vi "メイン.vi"() -> (2 "測定周期/ms":dbl, 3 "値転記用配列":T2[](array[typedef]))   [LabVIEW 2021] (continued)
                          # "csv作成の為表へクラスタ(実測値)書き込み"
                          # "⑤"
                          # "③"
                          # "④"
                          n2701 = local read "メインON/OFF_\n設定 10"() -> (w4992:T1)
                          n2702 = Unbundle By Name(w4992) -> ("使用ON/OFF"=w4988:bool)
                          n2703 = control-ref of="前回値転記用配列"() -> (w4986:refnum<vi>)
                          n2704 = local read "メイン設定_設定 10"() -> (w4993:T2)
                          n2705 = call "メイン_測定値配列_CSV転記サブ.vi"("メイン設定_設定入力"=w4993, "ループ反復数値入力"=w4990, "実測設定項目"=w4991, "使用ON/OFF"=w4988, "前回値転記用配列"=w4986) -> ("ループ反復数値出力"=w4989:i32, "メイン設定_設定出力"=w4987:T2)  [unwired: 5 in]
                          n2706 = local write "メイン設定_設定 10"(w4987) -> ()
                          n2707 = Add(x=11, y=w4989) -> (x+y=w4982:i32)
                          n2708 = Add(x=w4989, y=12) -> (x+y=w4980:i32)
                          n2709 = local read "csv作成表"() -> (w4976:string[][])
                          n2710 = Unbundle By Name(w4987) -> ("実測値(MAX)"=w4983:string, "実測値(MIN)"=w4984:string)
                          n2711 = Replace Array Subset(array=w4976, new element #1=w4983, index (row) #1=w4981, index (col) #1=w4982, new element #2=w4984, index (row) #2=w4981, index (col) #2=w4980) -> (w4978:string[][])
                          n2712 = Select(t=w4978, s=w4988, f=w4976) -> (s? t:f=w4979:string[][])
                          n2713 = local write "csv作成表"(w4979) -> ()
                        }
                        frame 10 {
                          w4999 = 2
                          # "B"
                          # "A"
                          # "csv作成の為表へクラスタ(実測値)書き込み"
                          # "⑤"
                          # "③"
                          # "④"
                          n2714 = local read "メインON/OFF_\n設定 11"() -> (w5010:T1)
                          n2715 = Unbundle By Name(w5010) -> ("使用ON/OFF"=w5006:bool)
                          n2716 = control-ref of="前回値転記用配列"() -> (w5004:refnum<vi>)
                          n2717 = local read "メイン設定_設定 11"() -> (w5011:T2)
                          n2718 = call "メイン_測定値配列_CSV転記サブ.vi"("メイン設定_設定入力"=w5011, "ループ反復数値入力"=w5008, "実測設定項目"=w5009, "使用ON/OFF"=w5006, "前回値転記用配列"=w5004) -> ("ループ反復数値出力"=w5007:i32, "メイン設定_設定出力"=w5005:T2)  [unwired: 5 in]
                          n2719 = local write "メイン設定_設定 11"(w5005) -> ()
                          n2720 = Add(x=12, y=w5007) -> (x+y=w5000:i32)
                          n2721 = Add(x=w5007, y=13) -> (x+y=w4998:i32)
                          n2722 = local read "csv作成表"() -> (w4994:string[][])
                          n2723 = Unbundle By Name(w5005) -> ("実測値(MAX)"=w5001:string, "実測値(MIN)"=w5002:string)
                          n2724 = Replace Array Subset(array=w4994, new element #1=w5001, index (row) #1=w4999, index (col) #1=w5000, new element #2=w5002, index (row) #2=w4999, index (col) #2=w4998) -> (w4996:string[][])
                          n2725 = Select(t=w4996, s=w5006, f=w4994) -> (s? t:f=w4997:string[][])
                          n2726 = local write "csv作成表"(w4997) -> ()
                        }
                        frame 11 {
                          w5017 = 2
                          # "B"
                          # "A"
                          # "csv作成の為表へクラスタ(実測値)書き込み"
                          # "⑤"
                          # "③"
                          # "④"
                          n2727 = local read "メインON/OFF_\n設定 12"() -> (w5028:T1)
                          n2728 = Unbundle By Name(w5028) -> ("使用ON/OFF"=w5024:bool)
                          n2729 = control-ref of="前回値転記用配列"() -> (w5022:refnum<vi>)
                          n2730 = local read "メイン設定_設定 12"() -> (w5029:T2)
                          n2731 = call "メイン_測定値配列_CSV転記サブ.vi"("メイン設定_設定入力"=w5029, "ループ反復数値入力"=w5026, "実測設定項目"=w5027, "使用ON/OFF"=w5024, "前回値転記用配列"=w5022) -> ("ループ反復数値出力"=w5025:i32, "メイン設定_設定出力"=w5023:T2)  [unwired: 5 in]
                          n2732 = local write "メイン設定_設定 12"(w5023) -> ()
                          n2733 = Add(x=13, y=w5025) -> (x+y=w5018:i32)
                          n2734 = Add(x=w5025, y=14) -> (x+y=w5016:i32)
                          n2735 = local read "csv作成表"() -> (w5012:string[][])
                          n2736 = Unbundle By Name(w5023) -> ("実測値(MAX)"=w5019:string, "実測値(MIN)"=w5020:string)
                          n2737 = Replace Array Subset(array=w5012, new element #1=w5019, index (row) #1=w5017, index (col) #1=w5018, new element #2=w5020, index (row) #2=w5017, index (col) #2=w5016) -> (w5014:string[][])
                          n2738 = Select(t=w5014, s=w5024, f=w5012) -> (s? t:f=w5015:string[][])
                          n2739 = local write "csv作成表"(w5015) -> ()
                        }
                      }
                    }
                  }
                }
                n2740 = local write "値転記用配列"(w4786) -> ()
                n2741 = flat-sequence {
                  tunnel: [w4801] -> w4787
                  tunnel: w4786 -> [w4801]
                  frame #0 {
                    w4796 = T9 {"Horizontal"=-51, "Vertical"=360} ("座標 5")
                    n2742 = control-ref of="このVI"() -> (w4797:refnum<vi>)
                    n2743 = property on="ペーン 2" class="Pane"("Origin"=w4796) -> ()  [unwired: 2 in, 2 out]
                    n2744 = property on="ペーン 2" class="Pane"("Origin"=w4796) -> ()  [unwired: 2 in, 2 out]
                    n2745 = control-ref of="このVI"() -> (w4799:refnum<vi>)
                    n2746 = Unbundle(w4796) -> ("Vertical"=w4798:i16)  [unwired: 1 out]
                    n2747 = Unbundle(w4796) -> ("Vertical"=w4800:i16)  [unwired: 1 out]
                    n2748 = call "メイン_装飾移動サブ.vi"("Y軸座標入力"=w4798, "VI入力"=w4797) -> ()  [unwired: 10 in]
                    n2749 = call "メイン_装飾枠移動サブ.vi"("Y軸座標入力"=w4800, "VI入力"=w4799) -> ()  [unwired: 10 in]
                  }
                }
              }
              frame #1 {
                w5031 = T8."Enabled" ("無効")
                # "⑪ボタンの無効解除"
                n2750 = for {
                  N: 12 -> [_]
                  tunnel: w5031 -> [w5034]
                  i -> [w5035]
                  n2751 = case shown="11" w5035 {
                    tunnel: w5034 -> [w5036 w5037 w5038 w5039 w5040 w5041 w5042 w5043 w5044 w5045 w5046 w5047]
                    frame 0, Default {
                      n2752 = property on="メイン測定ボタン_単発 1" class="Bool (指定)"("DisabledEnum"=w5036) -> ()  [unwired: 2 in, 2 out]
                      n2753 = property on="メイン測定ボタン_連続 1" class="Bool (指定)"("DisabledEnum"=w5036) -> ()  [unwired: 2 in, 2 out]
                    }
                    frame 1 {
                      n2754 = property on="メイン測定ボタン_単発 2" class="Bool (指定)"("DisabledEnum"=w5037) -> ()  [unwired: 2 in, 2 out]
                      n2755 = property on="メイン測定ボタン_連続 2" class="Bool (指定)"("DisabledEnum"=w5037) -> ()  [unwired: 2 in, 2 out]
                    }
                    frame 2 {
                      n2756 = property on="メイン測定ボタン_単発 3" class="Bool (指定)"("DisabledEnum"=w5038) -> ()  [unwired: 2 in, 2 out]
                      n2757 = property on="メイン測定ボタン_連続 3" class="Bool (指定)"("DisabledEnum"=w5038) -> ()  [unwired: 2 in, 2 out]
                    }
                    frame 3 {
                      n2758 = property on="メイン測定ボタン_単発 4" class="Bool (指定)"("DisabledEnum"=w5039) -> ()  [unwired: 2 in, 2 out]
                      n2759 = property on="メイン測定ボタン_連続 4" class="Bool (指定)"("DisabledEnum"=w5039) -> ()  [unwired: 2 in, 2 out]
                    }
                    frame 4 {
                      n2760 = property on="メイン測定ボタン_単発 5" class="Bool (指定)"("DisabledEnum"=w5040) -> ()  [unwired: 2 in, 2 out]
                      n2761 = property on="メイン測定ボタン_連続 5" class="Bool (指定)"("DisabledEnum"=w5040) -> ()  [unwired: 2 in, 2 out]
                    }
                    frame 5 {
                      n2762 = property on="メイン測定ボタン_連続 6" class="Bool (指定)"("DisabledEnum"=w5041) -> ()  [unwired: 2 in, 2 out]
                      n2763 = property on="メイン測定ボタン_単発 6" class="Bool (指定)"("DisabledEnum"=w5041) -> ()  [unwired: 2 in, 2 out]
                    }
                    frame 6 {
                      n2764 = property on="メイン測定ボタン_連続 7" class="Bool (指定)"("DisabledEnum"=w5042) -> ()  [unwired: 2 in, 2 out]
                      n2765 = property on="メイン測定ボタン_単発 7" class="Bool (指定)"("DisabledEnum"=w5042) -> ()  [unwired: 2 in, 2 out]
                    }
                    frame 7 {
                      n2766 = property on="メイン測定ボタン_単発 8" class="Bool (指定)"("DisabledEnum"=w5043) -> ()  [unwired: 2 in, 2 out]
                      n2767 = property on="メイン測定ボタン_連続 8" class="Bool (指定)"("DisabledEnum"=w5043) -> ()  [unwired: 2 in, 2 out]
                    }
                    frame 8 {
                      n2768 = property on="メイン測定ボタン_単発 9" class="Bool (指定)"("DisabledEnum"=w5044) -> ()  [unwired: 2 in, 2 out]
                      n2769 = property on="メイン測定ボタン_連続 9" class="Bool (指定)"("DisabledEnum"=w5044) -> ()  [unwired: 2 in, 2 out]
                    }
                    frame 9 {
                      n2770 = property on="メイン測定ボタン_単発 10" class="Bool (指定)"("DisabledEnum"=w5045) -> ()  [unwired: 2 in, 2 out]
                      n2771 = property on="メイン測定ボタン_連続 10" class="Bool (指定)"("DisabledEnum"=w5045) -> ()  [unwired: 2 in, 2 out]
                    }
                    frame 10 {
                      n2772 = property on="メイン測定ボタン_単発 11" class="Bool (指定)"("DisabledEnum"=w5046) -> ()  [unwired: 2 in, 2 out]
                      n2773 = property on="メイン測定ボタン_連続 11" class="Bool (指定)"("DisabledEnum"=w5046) -> ()  [unwired: 2 in, 2 out]
                    }
                    frame 11 {
                      n2774 = property on="メイン測定ボタン_連続 12" class="Bool (指定)"("DisabledEnum"=w5047) -> ()  [unwired: 2 in, 2 out]
                      n2775 = property on="メイン測定ボタン_単発 12" class="Bool (指定)"("DisabledEnum"=w5047) -> ()  [unwired: 2 in, 2 out]
                    }
                  }
                }
                n2776 = local write "測定新値\nリセット用 6"(TRUE) -> ()
                n2777 = property on="TOPページへ" class="Bool"("DisabledEnum"=w5031) -> ()  [unwired: 2 in, 2 out]
                n2778 = property on="保存して終了" class="Bool"("DisabledEnum"=w5031) -> ()  [unwired: 2 in, 2 out]
                n2779 = property on="保存せずに" class="Bool"("DisabledEnum"=w5031) -> ()  [unwired: 2 in, 2 out]
              }
            }
          }
          frame True {
          }
        }
      }
      frame "測定7" {
        # "⑦"
        # "項目別のボタンで測定を行う為、項目分必要"
        n2780 = local read "測定旧値 7"() -> (w5051:bool)
        n2781 = case shown="FALSE" w5051 {
          tunnel: w5049 -> [w5054 w5317]
          tunnel: [w5053 w5317] -> w5050
          frame False {
            n2782 = flat-sequence {
              tunnel: w5054 -> [w5064]
              tunnel: [w5056] -> w5052
              tunnel: [w5302] -> w5053
              tunnel: w5052 -> [w5302]
              frame #0 {
                # "※複製コピー時変更する項目\n①②\nローカル変数\n\n入れ子のケースストラクチャ\"2\"を複製\n\n0～数だけ変更する\n③④⑤\nローカル変数\n\n※AB\n行番号の変更をする必要がある\n\n--------------------------------\nこの後イベントストラクチャ複製する\n--------------------------------\nイベントストラクチャ複製後\n\n⑦⑧\nローカル変数\n⑨\n装飾体の位置設定\n-51は固定\n前ケースの数値+72\n⑩\n測定新値リセット用\nのボタンが複製されているので、\nフロントパネルを整理する\n⑪\nプロパティノード\nボタンの無効解除クリア以外全てのボタン対象"
                # "実測完了の簡易疑似コード\n\n1)測定モードが単発・連続、多点かで転記する配列を変える\n2)値転記用配列へ転記\n\nここからゲージ分を繰り返す必要がある\n\n3)配列0を取り出す\n4)配列0のポートNoを取り出す\n5)メイン測定_設定配列(測定1の対象配列)のポートNoと比較\n6)同じだったら処理をする。違ったら何もしない\n7)同じだったら配列0のメインON/OFF_設定1の使用ON/OFFがTrueかFalseか\nFlaseだったら前回値転記用配列から前回の値をメイン設定_設定へ転記\nTrueだったらメイン設定_設定の測定モードから\n0単発、1連続、3多点\nの処理を行う\n8)測定値をメイン設定_設定へ転記したら、前回転記用配列へ転記する"
                # "⑨"
                # "⑧"
                # "②"
                # "グループNO(表示上はポートNo)が同じだったら値を転記する\n\n測定した配列のグループNOと値転記用配列の他の指標グループNOを比較する\n＝だったら、対象の配列のON/OFFボタンがTrueか確認し、\nTrueだったら、測定モードによって、値かMAX、MINの数値を転記する\n\nグループNOが同じでなければ、転記しない(何もしない)"
                # "まず値転記用配列に測定の値を転記"
                # "実測定画面vi動作"
                n2783 = local read "メイン設定_設定 7"() -> (w5059:T2)
                n2784 = local read "測定新値 7"() -> (→"測定新値\nリセット用 7":bool)
                n2785 = local read "測定周期/ms"() -> (w5057:dbl)
                n2786 = Unbundle By Name(w5059) -> ("測定モード"=w5060:u16)
                n2787 = call "実測定画面.vi"("実測設定項目配列_\nメインからの転記"=w5064, "測定周期/ms_制御器"=w5057) -> ("実測設定項目配列_\nゲージIOへ転記用"=w5062:T2[], "実測設定項目配列_\n多点測定メイン転記用"=w5061:T2[])  [unwired: 11 in, 1 out]
                n2788 = case shown="1" w5060 {
                  tunnel: w5062 -> [w5071 w5072 _]
                  tunnel: [w5071 w5072 w5073] -> w5055
                  tunnel: w5061 -> [_ _ w5073]
                  frame 0, Default {
                  }
                  frame 1 {
                  }
                  frame 2 {
                  }
                }
                n2789 = for {
                  N: 32 -> [_]
                  tunnel: w5055 -> [w5080]
                  i -> [w5075]
                  # "①"
                  # "※複製コピーはこのケースで行う"
                  # "32回分"
                  # "比較する固定GNO"
                  n2790 = local read "メイン設定_設定 7"() -> (w5074:T2)
                  n2791 = Index Array(array=w5080, index=w5075) -> (element=w5079:T2)
                  n2792 = Unbundle By Name(w5074) -> ("ポートNo."=w5078:dbl)
                  n2793 = Unbundle By Name(w5079) -> ("ポートNo."=w5077:dbl)
                  n2794 = Equal?(x=w5078, y=w5077) -> (x = y?=w5076:bool)
                  n2795 = case shown="TRUE" w5076 {
                    tunnel: w5079 -> [_ w5082]
                    tunnel: w5075 -> [_ w5081]
                    frame False {
                    }
                    frame True {
                      n2796 = case shown="0, デフォルト" w5081 {
                        tunnel: w5082 -> [w5098 w5116 w5134 w5152 w5170 w5188 w5206 w5224 w5242 w5260 w5278 w5296]
                        tunnel: w5081 -> [w5097 w5115 w5133 w5151 w5169 w5187 w5205 w5223 w5241 w5259 w5277 w5295]
                        frame 0, Default {
                          w5088 = 2
                          # "B"
                          # "A"
                          # "csv作成の為表へクラスタ(実測値)書き込み"
                          # "⑤"
                          # "③"
                          # "④"
                          n2797 = local read "メインON/OFF_\n設定 1"() -> (w5099:T1)
                          n2798 = Unbundle By Name(w5099) -> ("使用ON/OFF"=w5095:bool)
                          n2799 = control-ref of="前回値転記用配列"() -> (w5093:refnum<vi>)
                          n2800 = local read "メイン設定_設定 1"() -> (w5100:T2)
                          n2801 = call "メイン_測定値配列_CSV転記サブ.vi"("メイン設定_設定入力"=w5100, "ループ反復数値入力"=w5097, "実測設定項目"=w5098, "使用ON/OFF"=w5095, "前回値転記用配列"=w5093) -> ("ループ反復数値出力"=w5096:i32, "メイン設定_設定出力"=w5094:T2)  [unwired: 5 in]
                          n2802 = local write "メイン設定_設定 1"(w5094) -> ()
                          n2803 = Add(x=2, y=w5096) -> (x+y=w5089:i32)
                          n2804 = Add(x=w5096, y=3) -> (x+y=w5087:i32)
                          n2805 = local read "csv作成表"() -> (w5083:string[][])
                          n2806 = Unbundle By Name(w5094) -> ("実測値(MAX)"=w5090:string, "実測値(MIN)"=w5091:string)
                          n2807 = Replace Array Subset(array=w5083, new element #1=w5090, index (row) #1=w5088, index (col) #1=w5089, new element #2=w5091, index (row) #2=w5088, index (col) #2=w5087) -> (w5085:string[][])
                          n2808 = Select(t=w5085, s=w5095, f=w5083) -> (s? t:f=w5086:string[][])
                          n2809 = local write "csv作成表"(w5086) -> ()
                        }
                        frame 1 {
                          w5106 = 2
                          # "B"
                          # "A"
                          # "csv作成の為表へクラスタ(実測値)書き込み"
                          # "⑤"
                          # "③"
                          # "④"
                          n2810 = local read "メインON/OFF_\n設定 2"() -> (w5117:T1)
                          n2811 = Unbundle By Name(w5117) -> ("使用ON/OFF"=w5113:bool)
                          n2812 = control-ref of="前回値転記用配列"() -> (w5111:refnum<vi>)
                          n2813 = local read "メイン設定_設定 2"() -> (w5118:T2)
                          n2814 = call "メイン_測定値配列_CSV転記サブ.vi"("メイン設定_設定入力"=w5118, "ループ反復数値入力"=w5115, "実測設定項目"=w5116, "使用ON/OFF"=w5113, "前回値転記用配列"=w5111) -> ("ループ反復数値出力"=w5114:i32, "メイン設定_設定出力"=w5112:T2)  [unwired: 5 in]
                          n2815 = local write "メイン設定_設定 2"(w5112) -> ()
                          n2816 = Add(x=3, y=w5114) -> (x+y=w5107:i32)
                          n2817 = Add(x=w5114, y=4) -> (x+y=w5105:i32)
                          n2818 = local read "csv作成表"() -> (w5101:string[][])
                          n2819 = Unbundle By Name(w5112) -> ("実測値(MAX)"=w5108:string, "実測値(MIN)"=w5109:string)
                          n2820 = Replace Array Subset(array=w5101, new element #1=w5108, index (row) #1=w5106, index (col) #1=w5107, new element #2=w5109, index (row) #2=w5106, index (col) #2=w5105) -> (w5103:string[][])
                          n2821 = Select(t=w5103, s=w5113, f=w5101) -> (s? t:f=w5104:string[][])
                          n2822 = local write "csv作成表"(w5104) -> ()
                        }
                        frame 2 {
                          w5124 = 2
                          # "B"
                          # "A"
                          # "csv作成の為表へクラスタ(実測値)書き込み"
                          # "⑤"
                          # "③"
                          # "④"
                          n2823 = local read "メインON/OFF_\n設定 3"() -> (w5135:T1)
                          n2824 = Unbundle By Name(w5135) -> ("使用ON/OFF"=w5131:bool)
                          n2825 = control-ref of="前回値転記用配列"() -> (w5129:refnum<vi>)
                          n2826 = local read "メイン設定_設定 3"() -> (w5136:T2)
                          n2827 = call "メイン_測定値配列_CSV転記サブ.vi"("メイン設定_設定入力"=w5136, "ループ反復数値入力"=w5133, "実測設定項目"=w5134, "使用ON/OFF"=w5131, "前回値転記用配列"=w5129) -> ("ループ反復数値出力"=w5132:i32, "メイン設定_設定出力"=w5130:T2)  [unwired: 5 in]
                          n2828 = local write "メイン設定_設定 3"(w5130) -> ()
                          n2829 = Add(x=4, y=w5132) -> (x+y=w5125:i32)
                          n2830 = Add(x=w5132, y=5) -> (x+y=w5123:i32)
                          n2831 = local read "csv作成表"() -> (w5119:string[][])
                          n2832 = Unbundle By Name(w5130) -> ("実測値(MAX)"=w5126:string, "実測値(MIN)"=w5127:string)
                          n2833 = Replace Array Subset(array=w5119, new element #1=w5126, index (row) #1=w5124, index (col) #1=w5125, new element #2=w5127, index (row) #2=w5124, index (col) #2=w5123) -> (w5121:string[][])
                          n2834 = Select(t=w5121, s=w5131, f=w5119) -> (s? t:f=w5122:string[][])
                          n2835 = local write "csv作成表"(w5122) -> ()
                        }
                        frame 3 {
                          w5142 = 2
                          # "B"
                          # "A"
                          # "csv作成の為表へクラスタ(実測値)書き込み"
                          # "⑤"
                          # "③"
                          # "④"
                          n2836 = local read "メインON/OFF_\n設定 4"() -> (w5153:T1)
                          n2837 = Unbundle By Name(w5153) -> ("使用ON/OFF"=w5149:bool)
                          n2838 = control-ref of="前回値転記用配列"() -> (w5147:refnum<vi>)
                          n2839 = local read "メイン設定_設定 4"() -> (w5154:T2)
                          n2840 = call "メイン_測定値配列_CSV転記サブ.vi"("メイン設定_設定入力"=w5154, "ループ反復数値入力"=w5151, "実測設定項目"=w5152, "使用ON/OFF"=w5149, "前回値転記用配列"=w5147) -> ("ループ反復数値出力"=w5150:i32, "メイン設定_設定出力"=w5148:T2)  [unwired: 5 in]
                          n2841 = local write "メイン設定_設定 4"(w5148) -> ()
                          n2842 = Add(x=5, y=w5150) -> (x+y=w5143:i32)
                          n2843 = Add(x=w5150, y=6) -> (x+y=w5141:i32)
                          n2844 = local read "csv作成表"() -> (w5137:string[][])
                          n2845 = Unbundle By Name(w5148) -> ("実測値(MAX)"=w5144:string, "実測値(MIN)"=w5145:string)
                          n2846 = Replace Array Subset(array=w5137, new element #1=w5144, index (row) #1=w5142, index (col) #1=w5143, new element #2=w5145, index (row) #2=w5142, index (col) #2=w5141) -> (w5139:string[][])
                          n2847 = Select(t=w5139, s=w5149, f=w5137) -> (s? t:f=w5140:string[][])
                          n2848 = local write "csv作成表"(w5140) -> ()
                        }
                        frame 4 {
                          w5160 = 2
                          # "B"
                          # "A"
                          # "csv作成の為表へクラスタ(実測値)書き込み"
                          # "⑤"
                          # "③"
                          # "④"
                          n2849 = local read "メインON/OFF_\n設定 5"() -> (w5171:T1)
                          n2850 = Unbundle By Name(w5171) -> ("使用ON/OFF"=w5167:bool)
                          n2851 = control-ref of="前回値転記用配列"() -> (w5165:refnum<vi>)
                          n2852 = local read "メイン設定_設定 5"() -> (w5172:T2)
                          n2853 = call "メイン_測定値配列_CSV転記サブ.vi"("メイン設定_設定入力"=w5172, "ループ反復数値入力"=w5169, "実測設定項目"=w5170, "使用ON/OFF"=w5167, "前回値転記用配列"=w5165) -> ("ループ反復数値出力"=w5168:i32, "メイン設定_設定出力"=w5166:T2)  [unwired: 5 in]
                          n2854 = local write "メイン設定_設定 5"(w5166) -> ()
                          n2855 = Add(x=6, y=w5168) -> (x+y=w5161:i32)
                          n2856 = Add(x=w5168, y=7) -> (x+y=w5159:i32)
                          n2857 = local read "csv作成表"() -> (w5155:string[][])
                          n2858 = Unbundle By Name(w5166) -> ("実測値(MAX)"=w5162:string, "実測値(MIN)"=w5163:string)
                          n2859 = Replace Array Subset(array=w5155, new element #1=w5162, index (row) #1=w5160, index (col) #1=w5161, new element #2=w5163, index (row) #2=w5160, index (col) #2=w5159) -> (w5157:string[][])
                          n2860 = Select(t=w5157, s=w5167, f=w5155) -> (s? t:f=w5158:string[][])
                          n2861 = local write "csv作成表"(w5158) -> ()
                        }
                        frame 5 {
                          w5178 = 2
                          # "B"
                          # "A"
                          # "csv作成の為表へクラスタ(実測値)書き込み"
                          # "⑤"
                          # "③"
                          # "④"
                          n2862 = local read "メインON/OFF_\n設定 6"() -> (w5189:T1)
                          n2863 = Unbundle By Name(w5189) -> ("使用ON/OFF"=w5185:bool)
                          n2864 = control-ref of="前回値転記用配列"() -> (w5183:refnum<vi>)
                          n2865 = local read "メイン設定_設定 6"() -> (w5190:T2)
                          n2866 = call "メイン_測定値配列_CSV転記サブ.vi"("メイン設定_設定入力"=w5190, "ループ反復数値入力"=w5187, "実測設定項目"=w5188, "使用ON/OFF"=w5185, "前回値転記用配列"=w5183) -> ("ループ反復数値出力"=w5186:i32, "メイン設定_設定出力"=w5184:T2)  [unwired: 5 in]
                          n2867 = local write "メイン設定_設定 6"(w5184) -> ()
                          n2868 = Add(x=7, y=w5186) -> (x+y=w5179:i32)
                          n2869 = Add(x=w5186, y=8) -> (x+y=w5177:i32)
                          n2870 = local read "csv作成表"() -> (w5173:string[][])
                          n2871 = Unbundle By Name(w5184) -> ("実測値(MAX)"=w5180:string, "実測値(MIN)"=w5181:string)
                          n2872 = Replace Array Subset(array=w5173, new element #1=w5180, index (row) #1=w5178, index (col) #1=w5179, new element #2=w5181, index (row) #2=w5178, index (col) #2=w5177) -> (w5175:string[][])
                          n2873 = Select(t=w5175, s=w5185, f=w5173) -> (s? t:f=w5176:string[][])
                          n2874 = local write "csv作成表"(w5176) -> ()
                        }
                        frame 6 {
                          w5196 = 2
                          # "B"
                          # "A"
                          # "csv作成の為表へクラスタ(実測値)書き込み"
                          # "⑤"
                          # "③"
                          # "④"
                          n2875 = local read "メインON/OFF_\n設定 7"() -> (w5207:T1)
                          n2876 = Unbundle By Name(w5207) -> ("使用ON/OFF"=w5203:bool)
                          n2877 = control-ref of="前回値転記用配列"() -> (w5201:refnum<vi>)
                          n2878 = local read "メイン設定_設定 7"() -> (w5208:T2)
                          n2879 = call "メイン_測定値配列_CSV転記サブ.vi"("メイン設定_設定入力"=w5208, "ループ反復数値入力"=w5205, "実測設定項目"=w5206, "使用ON/OFF"=w5203, "前回値転記用配列"=w5201) -> ("ループ反復数値出力"=w5204:i32, "メイン設定_設定出力"=w5202:T2)  [unwired: 5 in]
                          n2880 = local write "メイン設定_設定 7"(w5202) -> ()
                          n2881 = Add(x=8, y=w5204) -> (x+y=w5197:i32)
                          n2882 = Add(x=w5204, y=9) -> (x+y=w5195:i32)
                          n2883 = local read "csv作成表"() -> (w5191:string[][])
                          n2884 = Unbundle By Name(w5202) -> ("実測値(MAX)"=w5198:string, "実測値(MIN)"=w5199:string)
                          n2885 = Replace Array Subset(array=w5191, new element #1=w5198, index (row) #1=w5196, index (col) #1=w5197, new element #2=w5199, index (row) #2=w5196, index (col) #2=w5195) -> (w5193:string[][])
                          n2886 = Select(t=w5193, s=w5203, f=w5191) -> (s? t:f=w5194:string[][])
                          n2887 = local write "csv作成表"(w5194) -> ()
                        }
                        frame 7 {
                          w5214 = 2
                          # "B"
                          # "A"
                          # "csv作成の為表へクラスタ(実測値)書き込み"
                          # "⑤"
                          # "③"
                          # "④"
                          n2888 = local read "メインON/OFF_\n設定 8"() -> (w5225:T1)
                          n2889 = Unbundle By Name(w5225) -> ("使用ON/OFF"=w5221:bool)
                          n2890 = control-ref of="前回値転記用配列"() -> (w5219:refnum<vi>)
                          n2891 = local read "メイン設定_設定 8"() -> (w5226:T2)
                          n2892 = call "メイン_測定値配列_CSV転記サブ.vi"("メイン設定_設定入力"=w5226, "ループ反復数値入力"=w5223, "実測設定項目"=w5224, "使用ON/OFF"=w5221, "前回値転記用配列"=w5219) -> ("ループ反復数値出力"=w5222:i32, "メイン設定_設定出力"=w5220:T2)  [unwired: 5 in]
                          n2893 = local write "メイン設定_設定 8"(w5220) -> ()
                          n2894 = Add(x=9, y=w5222) -> (x+y=w5215:i32)
                          n2895 = Add(x=w5222, y=10) -> (x+y=w5213:i32)
                          n2896 = local read "csv作成表"() -> (w5209:string[][])
                          n2897 = Unbundle By Name(w5220) -> ("実測値(MAX)"=w5216:string, "実測値(MIN)"=w5217:string)
                          n2898 = Replace Array Subset(array=w5209, new element #1=w5216, index (row) #1=w5214, index (col) #1=w5215, new element #2=w5217, index (row) #2=w5214, index (col) #2=w5213) -> (w5211:string[][])
                          n2899 = Select(t=w5211, s=w5221, f=w5209) -> (s? t:f=w5212:string[][])
                          n2900 = local write "csv作成表"(w5212) -> ()
                        }
                        frame 8 {
                          w5232 = 2
                          # "B"
                          # "A"
                          # "csv作成の為表へクラスタ(実測値)書き込み"
                          # "⑤"
                          # "③"
                          # "④"
                          n2901 = local read "メインON/OFF_\n設定 9"() -> (w5243:T1)
                          n2902 = Unbundle By Name(w5243) -> ("使用ON/OFF"=w5239:bool)
                          n2903 = control-ref of="前回値転記用配列"() -> (w5237:refnum<vi>)
                          n2904 = local read "メイン設定_設定 9"() -> (w5244:T2)
                          n2905 = call "メイン_測定値配列_CSV転記サブ.vi"("メイン設定_設定入力"=w5244, "ループ反復数値入力"=w5241, "実測設定項目"=w5242, "使用ON/OFF"=w5239, "前回値転記用配列"=w5237) -> ("ループ反復数値出力"=w5240:i32, "メイン設定_設定出力"=w5238:T2)  [unwired: 5 in]
                          n2906 = local write "メイン設定_設定 9"(w5238) -> ()
                          n2907 = Add(x=10, y=w5240) -> (x+y=w5233:i32)
                          n2908 = Add(x=w5240, y=11) -> (x+y=w5231:i32)
                          n2909 = local read "csv作成表"() -> (w5227:string[][])
                          n2910 = Unbundle By Name(w5238) -> ("実測値(MAX)"=w5234:string, "実測値(MIN)"=w5235:string)
                          n2911 = Replace Array Subset(array=w5227, new element #1=w5234, index (row) #1=w5232, index (col) #1=w5233, new element #2=w5235, index (row) #2=w5232, index (col) #2=w5231) -> (w5229:string[][])
                          n2912 = Select(t=w5229, s=w5239, f=w5227) -> (s? t:f=w5230:string[][])
                          n2913 = local write "csv作成表"(w5230) -> ()
                        }
                        frame 9 {
                          w5250 = 2
                          # "B"
                          # "A"
                          # "csv作成の為表へクラスタ(実測値)書き込み"
                          # "⑤"
                          # "③"
                          # "④"
                          n2914 = local read "メインON/OFF_\n設定 10"() -> (w5261:T1)
                          n2915 = Unbundle By Name(w5261) -> ("使用ON/OFF"=w5257:bool)
                          n2916 = control-ref of="前回値転記用配列"() -> (w5255:refnum<vi>)
                          n2917 = local read "メイン設定_設定 10"() -> (w5262:T2)
                          n2918 = call "メイン_測定値配列_CSV転記サブ.vi"("メイン設定_設定入力"=w5262, "ループ反復数値入力"=w5259, "実測設定項目"=w5260, "使用ON/OFF"=w5257, "前回値転記用配列"=w5255) -> ("ループ反復数値出力"=w5258:i32, "メイン設定_設定出力"=w5256:T2)  [unwired: 5 in]
                          n2919 = local write "メイン設定_設定 10"(w5256) -> ()
                          n2920 = Add(x=11, y=w5258) -> (x+y=w5251:i32)
                          n2921 = Add(x=w5258, y=12) -> (x+y=w5249:i32)
                          n2922 = local read "csv作成表"() -> (w5245:string[][])
                          n2923 = Unbundle By Name(w5256) -> ("実測値(MAX)"=w5252:string, "実測値(MIN)"=w5253:string)
                          n2924 = Replace Array Subset(array=w5245, new element #1=w5252, index (row) #1=w5250, index (col) #1=w5251, new element #2=w5253, index (row) #2=w5250, index (col) #2=w5249) -> (w5247:string[][])
                          n2925 = Select(t=w5247, s=w5257, f=w5245) -> (s? t:f=w5248:string[][])
                          n2926 = local write "csv作成表"(w5248) -> ()
                        }
                        frame 10 {
                          w5268 = 2
                          # "B"
                          # "A"
                          # "csv作成の為表へクラスタ(実測値)書き込み"
                          # "⑤"
                          # "③"
                          # "④"
                          n2927 = local read "メインON/OFF_\n設定 11"() -> (w5279:T1)
                          n2928 = Unbundle By Name(w5279) -> ("使用ON/OFF"=w5275:bool)
                          n2929 = control-ref of="前回値転記用配列"() -> (w5273:refnum<vi>)
                          n2930 = local read "メイン設定_設定 11"() -> (w5280:T2)
                          n2931 = call "メイン_測定値配列_CSV転記サブ.vi"("メイン設定_設定入力"=w5280, "ループ反復数値入力"=w5277, "実測設定項目"=w5278, "使用ON/OFF"=w5275, "前回値転記用配列"=w5273) -> ("ループ反復数値出力"=w5276:i32, "メイン設定_設定出力"=w5274:T2)  [unwired: 5 in]
                          n2932 = local write "メイン設定_設定 11"(w5274) -> ()
                          n2933 = Add(x=12, y=w5276) -> (x+y=w5269:i32)
                          n2934 = Add(x=w5276, y=13) -> (x+y=w5267:i32)
                          n2935 = local read "csv作成表"() -> (w5263:string[][])
                          n2936 = Unbundle By Name(w5274) -> ("実測値(MAX)"=w5270:string, "実測値(MIN)"=w5271:string)
                          n2937 = Replace Array Subset(array=w5263, new element #1=w5270, index (row) #1=w5268, index (col) #1=w5269, new element #2=w5271, index (row) #2=w5268, index (col) #2=w5267) -> (w5265:string[][])
                          n2938 = Select(t=w5265, s=w5275, f=w5263) -> (s? t:f=w5266:string[][])
                          n2939 = local write "csv作成表"(w5266) -> ()
                        }
                        frame 11 {
                          w5286 = 2
                          # "B"
                          # "A"
                          # "csv作成の為表へクラスタ(実測値)書き込み"
                          # "⑤"
                          # "③"
                          # "④"
                          n2940 = local read "メインON/OFF_\n設定 12"() -> (w5297:T1)
                          n2941 = Unbundle By Name(w5297) -> ("使用ON/OFF"=w5293:bool)
                          n2942 = control-ref of="前回値転記用配列"() -> (w5291:refnum<vi>)
                          n2943 = local read "メイン設定_設定 12"() -> (w5298:T2)
                          n2944 = call "メイン_測定値配列_CSV転記サブ.vi"("メイン設定_設定入力"=w5298, "ループ反復数値入力"=w5295, "実測設定項目"=w5296, "使用ON/OFF"=w5293, "前回値転記用配列"=w5291) -> ("ループ反復数値出力"=w5294:i32, "メイン設定_設定出力"=w5292:T2)  [unwired: 5 in]
                          n2945 = local write "メイン設定_設定 12"(w5292) -> ()
                          n2946 = Add(x=13, y=w5294) -> (x+y=w5287:i32)
                          n2947 = Add(x=w5294, y=14) -> (x+y=w5285:i32)
                          n2948 = local read "csv作成表"() -> (w5281:string[][])
                          n2949 = Unbundle By Name(w5292) -> ("実測値(MAX)"=w5288:string, "実測値(MIN)"=w5289:string)
                          n2950 = Replace Array Subset(array=w5281, new element #1=w5288, index (row) #1=w5286, index (col) #1=w5287, new element #2=w5289, index (row) #2=w5286, index (col) #2=w5285) -> (w5283:string[][])
                          n2951 = Select(t=w5283, s=w5293, f=w5281) -> (s? t:f=w5284:string[][])
                          n2952 = local write "csv作成表"(w5284) -> ()
                        }
                      }
                    }
                  }
                }
                n2953 = local write "値転記用配列"(w5055) -> ()
                n2954 = flat-sequence {
                  tunnel: [w5070] -> w5056
                  tunnel: w5055 -> [w5070]
                  frame #0 {
                    w5065 = T9 {"Horizontal"=-51, "Vertical"=432} ("座標 6")
                    n2955 = control-ref of="このVI"() -> (w5066:refnum<vi>)
                    n2956 = property on="ペーン 2" class="Pane"("Origin"=w5065) -> ()  [unwired: 2 in, 2 out]
                    n2957 = property on="ペーン 2" class="Pane"("Origin"=w5065) -> ()  [unwired: 2 in, 2 out]
                    n2958 = control-ref of="このVI"() -> (w5068:refnum<vi>)
                    n2959 = Unbundle(w5065) -> ("Vertical"=w5067:i16)  [unwired: 1 out]
                    n2960 = Unbundle(w5065) -> ("Vertical"=w5069:i16)  [unwired: 1 out]
                    n2961 = call "メイン_装飾移動サブ.vi"("Y軸座標入力"=w5067, "VI入力"=w5066) -> ()  [unwired: 10 in]
                    n2962 = call "メイン_装飾枠移動サブ.vi"("Y軸座標入力"=w5069, "VI入力"=w5068) -> ()  [unwired: 10 in]
                  }
                }
              }
              frame #1 {
                w5300 = T8."Enabled" ("無効")
                # "⑪ボタンの無効解除"
                n2963 = local write "測定新値\nリセット用 7"(TRUE) -> ()
                n2964 = for {
                  N: 12 -> [_]
                  tunnel: w5300 -> [w5303]
                  i -> [w5304]
                  n2965 = case shown="11" w5304 {
                    tunnel: w5303 -> [w5305 w5306 w5307 w5308 w5309 w5310 w5311 w5312 w5313 w5314 w5315 w5316]
                    frame 0, Default {
                      n2966 = property on="メイン測定ボタン_単発 1" class="Bool (指定)"("DisabledEnum"=w5305) -> ()  [unwired: 2 in, 2 out]
                      n2967 = property on="メイン測定ボタン_連続 1" class="Bool (指定)"("DisabledEnum"=w5305) -> ()  [unwired: 2 in, 2 out]
                    }
                    frame 1 {
                      n2968 = property on="メイン測定ボタン_単発 2" class="Bool (指定)"("DisabledEnum"=w5306) -> ()  [unwired: 2 in, 2 out]
                      n2969 = property on="メイン測定ボタン_連続 2" class="Bool (指定)"("DisabledEnum"=w5306) -> ()  [unwired: 2 in, 2 out]
                    }
                    frame 2 {
                      n2970 = property on="メイン測定ボタン_単発 3" class="Bool (指定)"("DisabledEnum"=w5307) -> ()  [unwired: 2 in, 2 out]
                      n2971 = property on="メイン測定ボタン_連続 3" class="Bool (指定)"("DisabledEnum"=w5307) -> ()  [unwired: 2 in, 2 out]
                    }
                    frame 3 {
                      n2972 = property on="メイン測定ボタン_単発 4" class="Bool (指定)"("DisabledEnum"=w5308) -> ()  [unwired: 2 in, 2 out]
                      n2973 = property on="メイン測定ボタン_連続 4" class="Bool (指定)"("DisabledEnum"=w5308) -> ()  [unwired: 2 in, 2 out]
                    }
                    frame 4 {
                      n2974 = property on="メイン測定ボタン_単発 5" class="Bool (指定)"("DisabledEnum"=w5309) -> ()  [unwired: 2 in, 2 out]
                      n2975 = property on="メイン測定ボタン_連続 5" class="Bool (指定)"("DisabledEnum"=w5309) -> ()  [unwired: 2 in, 2 out]
                    }
                    frame 5 {
                      n2976 = property on="メイン測定ボタン_連続 6" class="Bool (指定)"("DisabledEnum"=w5310) -> ()  [unwired: 2 in, 2 out]
                      n2977 = property on="メイン測定ボタン_単発 6" class="Bool (指定)"("DisabledEnum"=w5310) -> ()  [unwired: 2 in, 2 out]
                    }
                    frame 6 {
                      n2978 = property on="メイン測定ボタン_連続 7" class="Bool (指定)"("DisabledEnum"=w5311) -> ()  [unwired: 2 in, 2 out]
                      n2979 = property on="メイン測定ボタン_単発 7" class="Bool (指定)"("DisabledEnum"=w5311) -> ()  [unwired: 2 in, 2 out]
                    }
                    frame 7 {
                      n2980 = property on="メイン測定ボタン_単発 8" class="Bool (指定)"("DisabledEnum"=w5312) -> ()  [unwired: 2 in, 2 out]
                      n2981 = property on="メイン測定ボタン_連続 8" class="Bool (指定)"("DisabledEnum"=w5312) -> ()  [unwired: 2 in, 2 out]
                    }
                    frame 8 {
                      n2982 = property on="メイン測定ボタン_単発 9" class="Bool (指定)"("DisabledEnum"=w5313) -> ()  [unwired: 2 in, 2 out]
                      n2983 = property on="メイン測定ボタン_連続 9" class="Bool (指定)"("DisabledEnum"=w5313) -> ()  [unwired: 2 in, 2 out]
                    }
                    frame 9 {
                      n2984 = property on="メイン測定ボタン_単発 10" class="Bool (指定)"("DisabledEnum"=w5314) -> ()  [unwired: 2 in, 2 out]
                      n2985 = property on="メイン測定ボタン_連続 10" class="Bool (指定)"("DisabledEnum"=w5314) -> ()  [unwired: 2 in, 2 out]
                    }
                    frame 10 {
                      n2986 = property on="メイン測定ボタン_単発 11" class="Bool (指定)"("DisabledEnum"=w5315) -> ()  [unwired: 2 in, 2 out]
                      n2987 = property on="メイン測定ボタン_連続 11" class="Bool (指定)"("DisabledEnum"=w5315) -> ()  [unwired: 2 in, 2 out]
                    }
                    frame 11 {
                      n2988 = property on="メイン測定ボタン_連続 12" class="Bool (指定)"("DisabledEnum"=w5316) -> ()  [unwired: 2 in, 2 out]
                      n2989 = property on="メイン測定ボタン_単発 12" class="Bool (指定)"("DisabledEnum"=w5316) -> ()  [unwired: 2 in, 2 out]
                    }
                  }
                }
                n2990 = property on="TOPページへ" class="Bool"("DisabledEnum"=w5300) -> ()  [unwired: 2 in, 2 out]
                n2991 = property on="保存して終了" class="Bool"("DisabledEnum"=w5300) -> ()  [unwired: 2 in, 2 out]
                n2992 = property on="保存せずに" class="Bool"("DisabledEnum"=w5300) -> ()  [unwired: 2 in, 2 out]
              }
            }
          }
          frame True {
          }
        }
      }
      frame "測定8" {
        # "⑦"
        # "項目別のボタンで測定を行う為、項目分必要"
        n2993 = local read "測定旧値 8"() -> (w5320:bool)
        n2994 = case shown="FALSE" w5320 {
          tunnel: w5318 -> [w5323 w5586]
          tunnel: [w5322 w5586] -> w5319
          frame False {
            n2995 = flat-sequence {
              tunnel: w5323 -> [w5333]
              tunnel: [w5325] -> w5321
              tunnel: [w5571] -> w5322
              tunnel: w5321 -> [w5571]
              frame #0 {
                # "※複製コピー時変更する項目\n①②\nローカル変数\n\n入れ子のケースストラクチャ\"2\"を複製\n\n0～数だけ変更する\n③④⑤\nローカル変数\n\n※AB\n行番号の変更をする必要がある\n\n--------------------------------\nこの後イベントストラクチャ複製する\n--------------------------------\nイベントストラクチャ複製後\n\n⑦⑧\nローカル変数\n⑨\n装飾体の位置設定\n-51は固定\n前ケースの数値+72\n⑩\n測定新値リセット用\nのボタンが複製されているので、\nフロントパネルを整理する\n⑪\nプロパティノード\nボタンの無効解除クリア以外全てのボタン対象"
                # "実測完了の簡易疑似コード\n\n1)測定モードが単発・連続、多点かで転記する配列を変える\n2)値転記用配列へ転記\n\nここからゲージ分を繰り返す必要がある\n\n3)配列0を取り出す\n4)配列0のポートNoを取り出す\n5)メイン測定_設定配列(測定1の対象配列)のポートNoと比較\n6)同じだったら処理をする。違ったら何もしない\n7)同じだったら配列0のメインON/OFF_設定1の使用ON/OFFがTrueかFalseか\nFlaseだったら前回値転記用配列から前回の値をメイン設定_設定へ転記\nTrueだったらメイン設定_設定の測定モードから\n0単発、1連続、3多点\nの処理を行う\n8)測定値をメイン設定_設定へ転記したら、前回転記用配列へ転記する"
                # "⑨"
                # "⑧"
                # "②"
                # "グループNO(表示上はポートNo)が同じだったら値を転記する\n\n測定した配列のグループNOと値転記用配列の他の指標グループNOを比較する\n＝だったら、対象の配列のON/OFFボタンがTrueか確認し、\nTrueだったら、測定モードによって、値かMAX、MINの数値を転記する\n\nグループNOが同じでなければ、転記しない(何もしない)"
                # "まず値転記用配列に測定の値を転記"
                # "実測定画面vi動作"
                n2996 = local read "メイン設定_設定 8"() -> (w5328:T2)
                n2997 = local read "測定新値 8"() -> (→"測定新値\nリセット用 8":bool)
                n2998 = local read "測定周期/ms"() -> (w5326:dbl)
                n2999 = Unbundle By Name(w5328) -> ("測定モード"=w5329:u16)
                n3000 = call "実測定画面.vi"("実測設定項目配列_\nメインからの転記"=w5333, "測定周期/ms_制御器"=w5326) -> ("実測設定項目配列_\nゲージIOへ転記用"=w5331:T2[], "実測設定項目配列_\n多点測定メイン転記用"=w5330:T2[])  [unwired: 11 in, 1 out]
                n3001 = case shown="1" w5329 {
                  tunnel: w5331 -> [w5340 w5341 _]
                  tunnel: [w5340 w5341 w5342] -> w5324
                  tunnel: w5330 -> [_ _ w5342]
                  frame 0, Default {
                  }
                  frame 1 {
                  }
                  frame 2 {
                  }
                }
                n3002 = for {
                  N: 32 -> [_]
                  tunnel: w5324 -> [w5349]
                  i -> [w5344]
                  # "①"
                  # "※複製コピーはこのケースで行う"
                  # "32回分"
                  # "比較する固定GNO"
                  n3003 = local read "メイン設定_設定 8"() -> (w5343:T2)
                  n3004 = Index Array(array=w5349, index=w5344) -> (element=w5348:T2)
                  n3005 = Unbundle By Name(w5343) -> ("ポートNo."=w5347:dbl)
                  n3006 = Unbundle By Name(w5348) -> ("ポートNo."=w5346:dbl)
                  n3007 = Equal?(x=w5347, y=w5346) -> (x = y?=w5345:bool)
                  n3008 = case shown="TRUE" w5345 {
                    tunnel: w5348 -> [_ w5351]
                    tunnel: w5344 -> [_ w5350]
                    frame False {
                    }
                    frame True {
                      n3009 = case shown="0, デフォルト" w5350 {
                        tunnel: w5351 -> [w5367 w5385 w5403 w5421 w5439 w5457 w5475 w5493 w5511 w5529 w5547 w5565]
                        tunnel: w5350 -> [w5366 w5384 w5402 w5420 w5438 w5456 w5474 w5492 w5510 w5528 w5546 w5564]
                        frame 0, Default {
                          w5357 = 2
                          # "B"
                          # "A"
                          # "csv作成の為表へクラスタ(実測値)書き込み"
                          # "⑤"
                          # "③"
                          # "④"
                          n3010 = local read "メインON/OFF_\n設定 1"() -> (w5368:T1)
                          n3011 = Unbundle By Name(w5368) -> ("使用ON/OFF"=w5364:bool)
                          n3012 = control-ref of="前回値転記用配列"() -> (w5362:refnum<vi>)
                          n3013 = local read "メイン設定_設定 1"() -> (w5369:T2)
                          n3014 = call "メイン_測定値配列_CSV転記サブ.vi"("メイン設定_設定入力"=w5369, "ループ反復数値入力"=w5366, "実測設定項目"=w5367, "使用ON/OFF"=w5364, "前回値転記用配列"=w5362) -> ("ループ反復数値出力"=w5365:i32, "メイン設定_設定出力"=w5363:T2)  [unwired: 5 in]
                          n3015 = local write "メイン設定_設定 1"(w5363) -> ()
                          n3016 = Add(x=2, y=w5365) -> (x+y=w5358:i32)
                          n3017 = Add(x=w5365, y=3) -> (x+y=w5356:i32)
                          n3018 = local read "csv作成表"() -> (w5352:string[][])
                          n3019 = Unbundle By Name(w5363) -> ("実測値(MAX)"=w5359:string, "実測値(MIN)"=w5360:string)
                          n3020 = Replace Array Subset(array=w5352, new element #1=w5359, index (row) #1=w5357, index (col) #1=w5358, new element #2=w5360, index (row) #2=w5357, index (col) #2=w5356) -> (w5354:string[][])
                          n3021 = Select(t=w5354, s=w5364, f=w5352) -> (s? t:f=w5355:string[][])
                          n3022 = local write "csv作成表"(w5355) -> ()
                        }
                        frame 1 {
                          w5375 = 2
                          # "B"
                          # "A"
                          # "csv作成の為表へクラスタ(実測値)書き込み"
                          # "⑤"
                          # "③"
                          # "④"
                          n3023 = local read "メインON/OFF_\n設定 2"() -> (w5386:T1)
                          n3024 = Unbundle By Name(w5386) -> ("使用ON/OFF"=w5382:bool)
                          n3025 = control-ref of="前回値転記用配列"() -> (w5380:refnum<vi>)
                          n3026 = local read "メイン設定_設定 2"() -> (w5387:T2)
                          n3027 = call "メイン_測定値配列_CSV転記サブ.vi"("メイン設定_設定入力"=w5387, "ループ反復数値入力"=w5384, "実測設定項目"=w5385, "使用ON/OFF"=w5382, "前回値転記用配列"=w5380) -> ("ループ反復数値出力"=w5383:i32, "メイン設定_設定出力"=w5381:T2)  [unwired: 5 in]
                          n3028 = local write "メイン設定_設定 2"(w5381) -> ()
                          n3029 = Add(x=3, y=w5383) -> (x+y=w5376:i32)
                          n3030 = Add(x=w5383, y=4) -> (x+y=w5374:i32)
                          n3031 = local read "csv作成表"() -> (w5370:string[][])
                          n3032 = Unbundle By Name(w5381) -> ("実測値(MAX)"=w5377:string, "実測値(MIN)"=w5378:string)
                          n3033 = Replace Array Subset(array=w5370, new element #1=w5377, index (row) #1=w5375, index (col) #1=w5376, new element #2=w5378, index (row) #2=w5375, index (col) #2=w5374) -> (w5372:string[][])
                          n3034 = Select(t=w5372, s=w5382, f=w5370) -> (s? t:f=w5373:string[][])
                          n3035 = local write "csv作成表"(w5373) -> ()
                        }
                        frame 2 {
                          w5393 = 2
                          # "B"
                          # "A"
                          # "csv作成の為表へクラスタ(実測値)書き込み"
                          # "⑤"
                          # "③"
                          # "④"
                          n3036 = local read "メインON/OFF_\n設定 3"() -> (w5404:T1)
                          n3037 = Unbundle By Name(w5404) -> ("使用ON/OFF"=w5400:bool)
                          n3038 = control-ref of="前回値転記用配列"() -> (w5398:refnum<vi>)
                          n3039 = local read "メイン設定_設定 3"() -> (w5405:T2)
                          n3040 = call "メイン_測定値配列_CSV転記サブ.vi"("メイン設定_設定入力"=w5405, "ループ反復数値入力"=w5402, "実測設定項目"=w5403, "使用ON/OFF"=w5400, "前回値転記用配列"=w5398) -> ("ループ反復数値出力"=w5401:i32, "メイン設定_設定出力"=w5399:T2)  [unwired: 5 in]
                          n3041 = local write "メイン設定_設定 3"(w5399) -> ()
                          n3042 = Add(x=4, y=w5401) -> (x+y=w5394:i32)
                          n3043 = Add(x=w5401, y=5) -> (x+y=w5392:i32)
                          n3044 = local read "csv作成表"() -> (w5388:string[][])
                          n3045 = Unbundle By Name(w5399) -> ("実測値(MAX)"=w5395:string, "実測値(MIN)"=w5396:string)
                          n3046 = Replace Array Subset(array=w5388, new element #1=w5395, index (row) #1=w5393, index (col) #1=w5394, new element #2=w5396, index (row) #2=w5393, index (col) #2=w5392) -> (w5390:string[][])
                          n3047 = Select(t=w5390, s=w5400, f=w5388) -> (s? t:f=w5391:string[][])
                          n3048 = local write "csv作成表"(w5391) -> ()
                        }
                        frame 3 {
                          w5411 = 2
                          # "B"
                          # "A"
                          # "csv作成の為表へクラスタ(実測値)書き込み"
                          # "⑤"
                          # "③"
                          # "④"
                          n3049 = local read "メインON/OFF_\n設定 4"() -> (w5422:T1)
                          n3050 = Unbundle By Name(w5422) -> ("使用ON/OFF"=w5418:bool)
                          n3051 = control-ref of="前回値転記用配列"() -> (w5416:refnum<vi>)
                          n3052 = local read "メイン設定_設定 4"() -> (w5423:T2)
                          n3053 = call "メイン_測定値配列_CSV転記サブ.vi"("メイン設定_設定入力"=w5423, "ループ反復数値入力"=w5420, "実測設定項目"=w5421, "使用ON/OFF"=w5418, "前回値転記用配列"=w5416) -> ("ループ反復数値出力"=w5419:i32, "メイン設定_設定出力"=w5417:T2)  [unwired: 5 in]
                          n3054 = local write "メイン設定_設定 4"(w5417) -> ()
                          n3055 = Add(x=5, y=w5419) -> (x+y=w5412:i32)
                          n3056 = Add(x=w5419, y=6) -> (x+y=w5410:i32)
                          n3057 = local read "csv作成表"() -> (w5406:string[][])
                          n3058 = Unbundle By Name(w5417) -> ("実測値(MAX)"=w5413:string, "実測値(MIN)"=w5414:string)
                          n3059 = Replace Array Subset(array=w5406, new element #1=w5413, index (row) #1=w5411, index (col) #1=w5412, new element #2=w5414, index (row) #2=w5411, index (col) #2=w5410) -> (w5408:string[][])
                          n3060 = Select(t=w5408, s=w5418, f=w5406) -> (s? t:f=w5409:string[][])
                          n3061 = local write "csv作成表"(w5409) -> ()
                        }
                        frame 4 {
                          w5429 = 2
                          # "B"
                          # "A"
                          # "csv作成の為表へクラスタ(実測値)書き込み"
                          # "⑤"
                          # "③"
                          # "④"
                          n3062 = local read "メインON/OFF_\n設定 5"() -> (w5440:T1)
                          n3063 = Unbundle By Name(w5440) -> ("使用ON/OFF"=w5436:bool)
                          n3064 = control-ref of="前回値転記用配列"() -> (w5434:refnum<vi>)
                          n3065 = local read "メイン設定_設定 5"() -> (w5441:T2)
                          n3066 = call "メイン_測定値配列_CSV転記サブ.vi"("メイン設定_設定入力"=w5441, "ループ反復数値入力"=w5438, "実測設定項目"=w5439, "使用ON/OFF"=w5436, "前回値転記用配列"=w5434) -> ("ループ反復数値出力"=w5437:i32, "メイン設定_設定出力"=w5435:T2)  [unwired: 5 in]
                          n3067 = local write "メイン設定_設定 5"(w5435) -> ()
                          n3068 = Add(x=6, y=w5437) -> (x+y=w5430:i32)
                          n3069 = Add(x=w5437, y=7) -> (x+y=w5428:i32)
                          n3070 = local read "csv作成表"() -> (w5424:string[][])
                          n3071 = Unbundle By Name(w5435) -> ("実測値(MAX)"=w5431:string, "実測値(MIN)"=w5432:string)
                          n3072 = Replace Array Subset(array=w5424, new element #1=w5431, index (row) #1=w5429, index (col) #1=w5430, new element #2=w5432, index (row) #2=w5429, index (col) #2=w5428) -> (w5426:string[][])
                          n3073 = Select(t=w5426, s=w5436, f=w5424) -> (s? t:f=w5427:string[][])
                          n3074 = local write "csv作成表"(w5427) -> ()
                        }
                        frame 5 {
                          w5447 = 2
                          # "B"
                          # "A"
                          # "csv作成の為表へクラスタ(実測値)書き込み"
                          # "⑤"
                          # "③"
                          # "④"
                          n3075 = local read "メインON/OFF_\n設定 6"() -> (w5458:T1)
                          n3076 = Unbundle By Name(w5458) -> ("使用ON/OFF"=w5454:bool)
                          n3077 = control-ref of="前回値転記用配列"() -> (w5452:refnum<vi>)
                          n3078 = local read "メイン設定_設定 6"() -> (w5459:T2)
                          n3079 = call "メイン_測定値配列_CSV転記サブ.vi"("メイン設定_設定入力"=w5459, "ループ反復数値入力"=w5456, "実測設定項目"=w5457, "使用ON/OFF"=w5454, "前回値転記用配列"=w5452) -> ("ループ反復数値出力"=w5455:i32, "メイン設定_設定出力"=w5453:T2)  [unwired: 5 in]
                          n3080 = local write "メイン設定_設定 6"(w5453) -> ()
                          n3081 = Add(x=7, y=w5455) -> (x+y=w5448:i32)
                          n3082 = Add(x=w5455, y=8) -> (x+y=w5446:i32)
                          n3083 = local read "csv作成表"() -> (w5442:string[][])
                          n3084 = Unbundle By Name(w5453) -> ("実測値(MAX)"=w5449:string, "実測値(MIN)"=w5450:string)
                          n3085 = Replace Array Subset(array=w5442, new element #1=w5449, index (row) #1=w5447, index (col) #1=w5448, new element #2=w5450, index (row) #2=w5447, index (col) #2=w5446) -> (w5444:string[][])
                          n3086 = Select(t=w5444, s=w5454, f=w5442) -> (s? t:f=w5445:string[][])
                          n3087 = local write "csv作成表"(w5445) -> ()
                        }
                        frame 6 {
                          w5465 = 2
                          # "B"
                          # "A"
                          # "csv作成の為表へクラスタ(実測値)書き込み"
                          # "⑤"
                          # "③"
                          # "④"
                          n3088 = local read "メインON/OFF_\n設定 7"() -> (w5476:T1)
                          n3089 = Unbundle By Name(w5476) -> ("使用ON/OFF"=w5472:bool)
                          n3090 = control-ref of="前回値転記用配列"() -> (w5470:refnum<vi>)
                          n3091 = local read "メイン設定_設定 7"() -> (w5477:T2)
                          n3092 = call "メイン_測定値配列_CSV転記サブ.vi"("メイン設定_設定入力"=w5477, "ループ反復数値入力"=w5474, "実測設定項目"=w5475, "使用ON/OFF"=w5472, "前回値転記用配列"=w5470) -> ("ループ反復数値出力"=w5473:i32, "メイン設定_設定出力"=w5471:T2)  [unwired: 5 in]
                          n3093 = local write "メイン設定_設定 7"(w5471) -> ()
                          n3094 = Add(x=8, y=w5473) -> (x+y=w5466:i32)
                          n3095 = Add(x=w5473, y=9) -> (x+y=w5464:i32)
                          n3096 = local read "csv作成表"() -> (w5460:string[][])
                          n3097 = Unbundle By Name(w5471) -> ("実測値(MAX)"=w5467:string, "実測値(MIN)"=w5468:string)
                          n3098 = Replace Array Subset(array=w5460, new element #1=w5467, index (row) #1=w5465, index (col) #1=w5466, new element #2=w5468, index (row) #2=w5465, index (col) #2=w5464) -> (w5462:string[][])
                          n3099 = Select(t=w5462, s=w5472, f=w5460) -> (s? t:f=w5463:string[][])
                          n3100 = local write "csv作成表"(w5463) -> ()
                        }
                        frame 7 {
                          w5483 = 2
                          # "B"
                          # "A"
                          # "csv作成の為表へクラスタ(実測値)書き込み"
                          # "⑤"
                          # "③"
                          # "④"
                          n3101 = local read "メインON/OFF_\n設定 8"() -> (w5494:T1)
                          n3102 = Unbundle By Name(w5494) -> ("使用ON/OFF"=w5490:bool)
                          n3103 = control-ref of="前回値転記用配列"() -> (w5488:refnum<vi>)
                          n3104 = local read "メイン設定_設定 8"() -> (w5495:T2)
                          n3105 = call "メイン_測定値配列_CSV転記サブ.vi"("メイン設定_設定入力"=w5495, "ループ反復数値入力"=w5492, "実測設定項目"=w5493, "使用ON/OFF"=w5490, "前回値転記用配列"=w5488) -> ("ループ反復数値出力"=w5491:i32, "メイン設定_設定出力"=w5489:T2)  [unwired: 5 in]
                          n3106 = local write "メイン設定_設定 8"(w5489) -> ()
                          n3107 = Add(x=9, y=w5491) -> (x+y=w5484:i32)
